vi "Launch Icon Editor From String.vi"(8 "error in (no error)":errorcluster, 11 "Flattened Icon.lvclass in":string) -> (0 "error out":errorcluster, 3 "Flattened Icon.lvclass out":string, 4 "Canceled?":bool)   [LabVIEW 2020]
uses:
  lv_icon.vi
  vi.lib/LabVIEW Icon API/lv_icon/lv_icon.lvlib
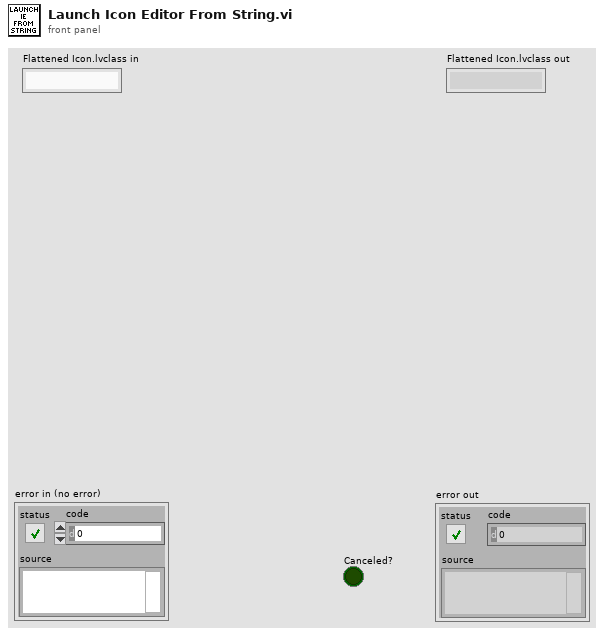
[diagram p1: front panel]
types:
  T1 = enum32{"Invalid", "Standard", "Closed", "Hidden", "Minimized", "Maximized"}
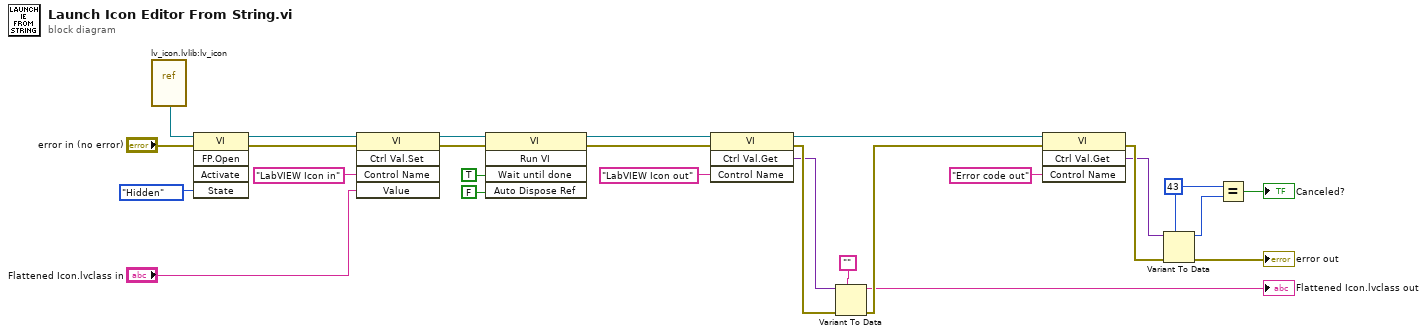
[diagram p0: block diagram]
diagram:
  w7 = 43 ("y")
  n1 = vi-ref "lv_icon.lvlib:lv_icon.vi"() -> (w27:refnum<vi>)
  n2 = invoke class="VI" method="FP.Open"(reference=w27, error in="error in (no error)", "State"=T1."Hidden") -> (reference out=w6:refnum<vi>, error out=w25:errorcluster)  [unwired: 2 in, 3 out]
  n3 = invoke class="VI" method="Ctrl Val.Set"(reference=w6, error in=w25, "Control Name"="LabVIEW Icon in", "Value"="Flattened Icon.lvclass in") -> (reference out=w22:refnum<vi>, error out=w23:errorcluster)  [unwired: 1 in, 3 out]
  n4 = invoke class="VI" method="Run VI"(reference=w22, error in=w23, "Wait until done"=TRUE ("Wait Until Done"), "Auto Dispose Ref"=FALSE ("Auto Dispose Reference")) -> (reference out=w18:refnum<vi>, error out=w17:errorcluster)  [unwired: 1 in, 3 out]
  n5 = invoke class="VI" method="Ctrl Val.Get"(reference=w18, error in=w17, "Control Name"="LabVIEW Icon out") -> (reference out=w9:refnum<vi>, error out=w11:errorcluster, "Get Control Value Variant"=w10:variant)  [unwired: 1 in, 1 out]
  n6 = Variant To Data(error in=w11, type="", Variant=w10) -> (data=→"Flattened Icon.lvclass out":string, error out=w4:errorcluster)
  n7 = invoke class="VI" method="Ctrl Val.Get"(reference=w9, error in=w4, "Control Name"="Error code out") -> (error out=w15:errorcluster, "Get Control Value Variant"=w14:variant)  [unwired: 1 in, 2 out]
  n8 = Variant To Data(error in=w15, type=w7, Variant=w14) -> (data=w13:i32, error out=→"error out":errorcluster)
  n9 = Equal?(x=w7, y=w13) -> (x = y?=→"Canceled?":bool)
